vi "Pulse Generator.vi"(3 "Reset Counter":bool, 5 "Terminal Count?":bool, 6 "High Pulse Time":u32=1000) -> (0 "Reset State":bool, 2 "CtrOut":bool)   [LabVIEW 2010]
doc: "This VI generates a pulse signal whenever the specified terminal count is reached with the high state determined by the \"High Pulse Time (us)\" value."
uses:
  <userlib>/_NI VeriStand FPGA Support/NI VeriStand RIO Library/IP Based IO/Counter/common/Pulse State.ctl
panel:
  out "Pulse State":T1
  out "Tick Counter":u32
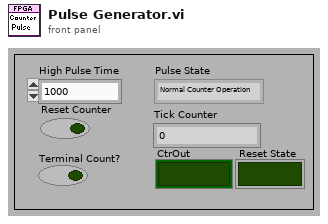
[diagram p1: front panel]
types:
  T1 = typedef "Pulse State.ctl" = enum16{"Normal Counter Operation", "Start Pulse Generation", "End Pulse Generation"}
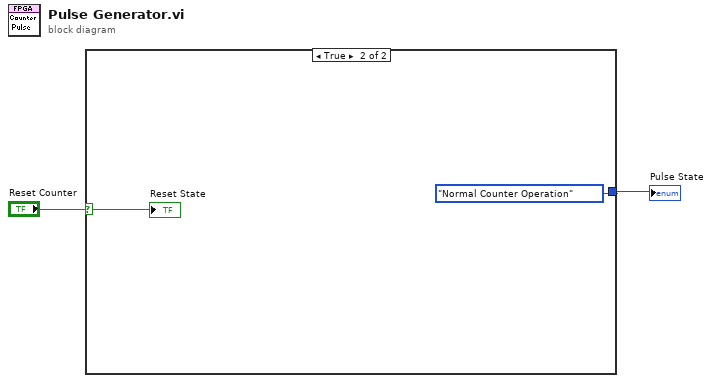
[diagram p0: block diagram]
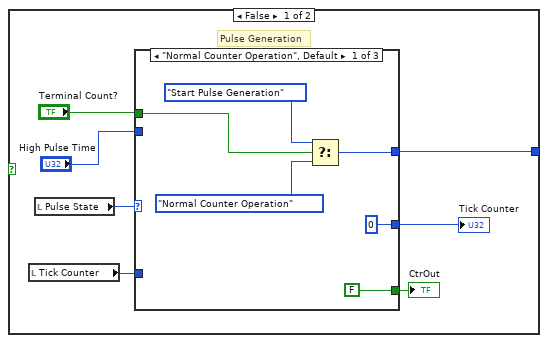
[diagram p2: hidden frame]
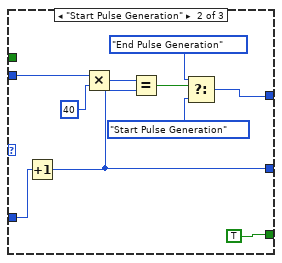
[diagram p3: hidden frame]
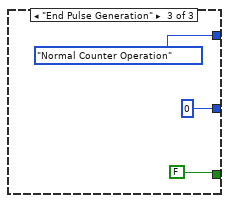
[diagram p4: hidden frame]
diagram:
  n1 = case shown="True" "Reset Counter" {
    selector: "Reset Counter" -> [_ w29]
    tunnel: [w4 Pulse_State."Normal Counter Operation" ("Enum")] -> w2
    frame False {
      # "Pulse Generation"
      n2 = local read "Tick Counter"() -> (w7:u32)
      n3 = local read "Pulse State"() -> (w3:T1)
      n4 = case shown="\"Normal Counter Operation\", Default" w3 {
        tunnel: [w13 w19 Pulse_State."Normal Counter Operation" ("Enum")] -> w4
        tunnel: [FALSE TRUE ("DIO2") FALSE ("DIO2")] -> w5
        tunnel: w7 -> [_ w24 _]
        tunnel: [u32 0 w23 u32 0] -> w8
        tunnel: "Terminal Count?" -> [w10 _ _]
        tunnel: "High Pulse Time" -> [_ w16 _]
        frame "Normal Counter Operation", Default {
          n5 = Select(t=Pulse_State."Start Pulse Generation" ("Enum"), s=w10, f=Pulse_State."Normal Counter Operation" ("Enum")) -> (s? t:f=w13:T1)
        }
        frame "Start Pulse Generation" {
          n6 = Increment(x=w24) -> (x+1=w23:u32)
          n7 = Multiply(x=w16, y=u32 40 ("x+1")) -> (x*y=w18:u32)
          n8 = Equal?(x=w18, y=w23) -> (x = y?=w22:bool)
          n9 = Select(t=Pulse_State."End Pulse Generation" ("Enum"), s=w22, f=Pulse_State."Start Pulse Generation" ("Enum")) -> (s? t:f=w19:T1)
        }
        frame "End Pulse Generation" {
        }
      }
      "Tick Counter" <- w8
      "CtrOut" <- w5
    }
    frame True {
      "Reset State" <- w29
    }
  }
  "Pulse State" <- w2
